vi "Create_New_Build.vi"(8 "error in (no error)":errorcluster, 9 "buildObject":T1, 11 "Build in":refnum<class "AB_Build.lvclass">) -> (0 "error out":errorcluster, 3 "Build out":refnum<class "AB_Build.lvclass">)   [LabVIEW 2020, in "AB_Deployment.lvlib"]
uses:
  <vilib>/AppBuilder/AB_Classes/Deployment/AB_Deployment.lvlib
  <vilib>/AppBuilder/AB_Classes/Build/AB_Build.lvclass
  <resource>/Framework/Providers/API/ItemRef.ctl
  <resource>/Framework/Providers/Common/provcom_StringGlobals.vi
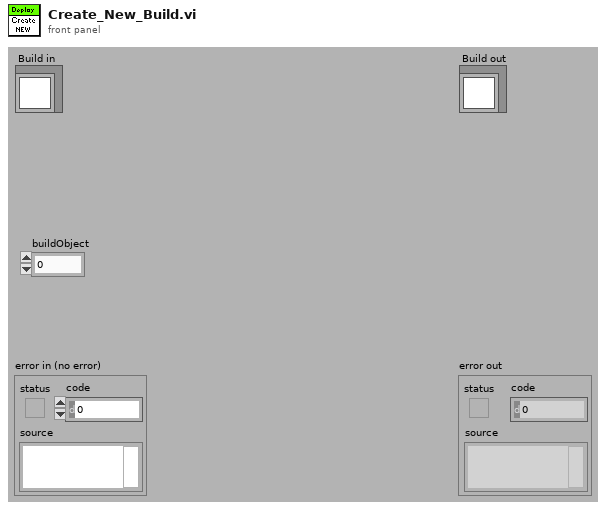
[diagram p1: front panel]
types:
  T1 = typedef "ItemRef.ctl" = u64
  T2 = typedef "AB_Build.ctl" = cluster{"buildSpecName":string, "buildSpecDescription":string, "destinations":refnum<class "AB_Destination.lvclass">[], "exclusionOption":T3, "defaultLanguage":string, "supportedLanguages":string[], "excludedDirectories":path[], "buildContext":refnum<vi>, "buildObject":T1, "preview":bool, "programatic":bool, "progressBarEvents":T4, "userLog_Path":path, "preActionID":string, "preAction_Path":path, "postActionID":string, "postAction_Path":path, "eng_checkForBrokenVIs?":bool, "eng_verboseLinkerErrors?":bool, "localDest_Path":path, "targetDest_Path":path, "removeVIObject":u16, "cache":refnum<class "PreviewCache.lvclass">, "use cache":bool, "previewCache_ID":string, "buildCache_ID":string, "eng_TempLocalDest_Path":path, "eng_collectDependencies?":bool, "versionInfo":cluster{"buildVersion":cluster{"major":u16, "minor":u16, "patch":u16, "build":u16}, "autoIncrement":bool}, "eng_enableVIChecksums":bool}
  T3 = typedef "AB_Exclusion_Option.ctl" = cluster{"typedefs":bool, "polymorphicVIs":bool, "unusedLibraryItems":bool, "modifyLibraryFile":bool, "edit-timeDependencies":bool, "inlineVIs":bool, "dependent PPLs":bool, "dependent DLLs":bool}
  T4 = typedef "provcom_ProgressBar_Events.ctl" = cluster{"newJob":refnum<user-event>, "newItem":refnum<user-event>, "errorMsg":T5, "cancel":refnum<user-event>}
  T5 = typedef "mxLvBuildError.ctl" = refnum<user-event>
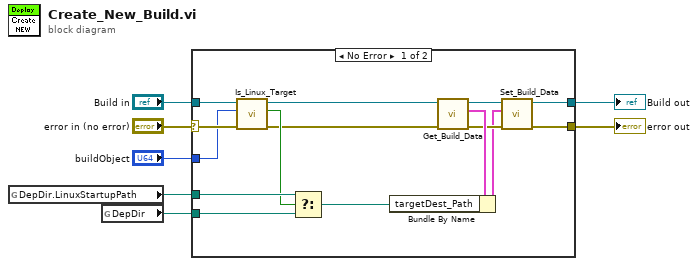
[diagram p0: block diagram]
diagram:
  n1 = global read "provcom_StringGlobals.vi" "DepDir.LinuxStartupPath"() -> (w1:path)
  n2 = global read "provcom_StringGlobals.vi" "DepDir"() -> (w2:path)
  n3 = case shown="No Error" "error in (no error)" {
    selector: "error in (no error)" -> [w17 w23]
    tunnel: "buildObject" -> [w16 _]
    tunnel: "Build in" -> [w18 w24]
    tunnel: [w9 w23] -> w5
    tunnel: [w11 w24] -> w4
    tunnel: w2 -> [w14 _]
    tunnel: w1 -> [w15 _]
    frame No Error {
      n4 = call <vilib>:"Is_Linux_Target.vi"("error in (no error)"=w17, "buildObject"=w16, "AB_Build in"=w18) -> ("error out"=w10:errorcluster, "Linux?"=w13:bool, "AB_Build out"=w12:refnum<class "AB_Build.lvclass">)  [unwired: 6 in]
      n5 = Select(t=w15, s=w13, f=w14) -> (s? t:f=w8:path)
      n6 = call <vilib>:"Get_Build_Data.vi"("error in (no error)"=w10, "Class in"=w12) -> ("error out"=w20:errorcluster, "data"=w22:T2, "Class out"=w21:refnum<class "AB_Build.lvclass">)  [unwired: 7 out]
      n7 = Bundle By Name(cluster=w22, "targetDest_Path"=w8) -> (w19:T2)
      n8 = call <vilib>:"Set_Build_Data.vi"("error in (no error)"=w20, "data"=w19, "Class in"=w21) -> ("error out"=w9:errorcluster, "Class out"=w11:refnum<class "AB_Build.lvclass">)  [unwired: 7 out]
    }
    frame Error {
    }
  }
  "error out" <- w5
  "Build out" <- w4
